vi "SCM1 He level field control.vi"() -> ()   [LabVIEW 2025]
panel:
  out "Waveform Chart":waveform(dbl)(graph)
  in  "level watch dog":bool
  in  "port number":u16=3363
  out "error out":errorcluster
  in  "Data mac ip address":string="146.201.236.102"
  out "low level":bool
  # "Import LHe level from a VI (SCM1 He level.vi) that communicates with the LHe level meter.\nDue to previous issues with communicaiton with the LHe level meter, the SCM1 He level.vi is running in \na separate computer. \nIf the He level is reported to be low, this VI abort some VI's and set the field to zero."
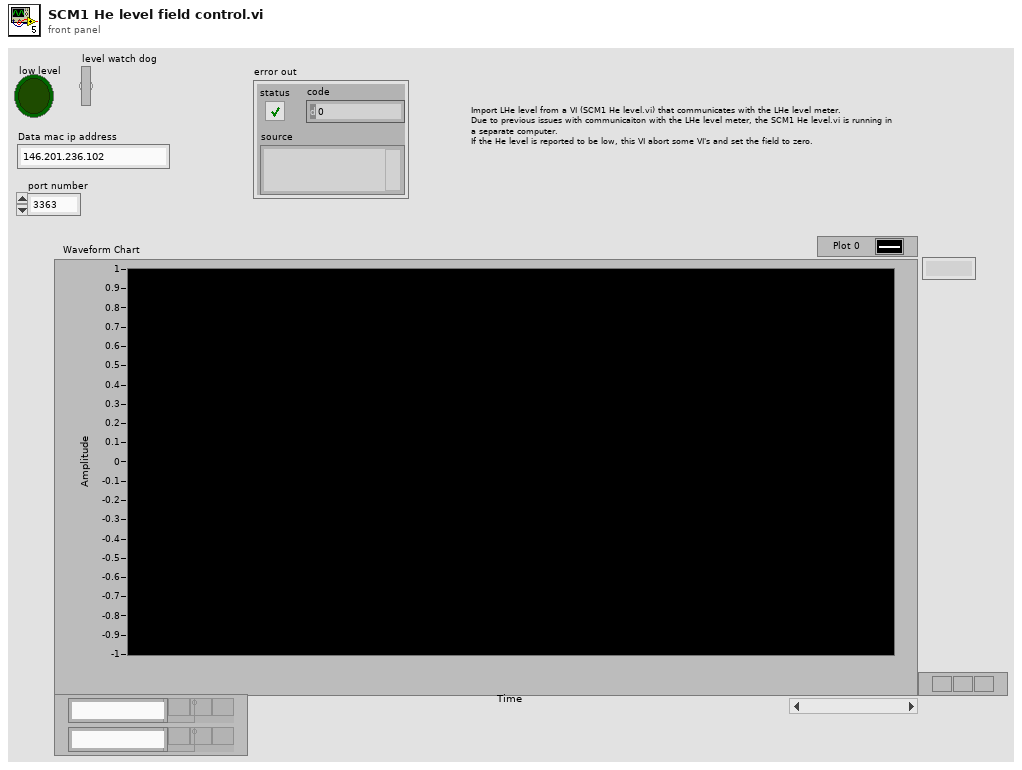
[diagram p1: front panel]
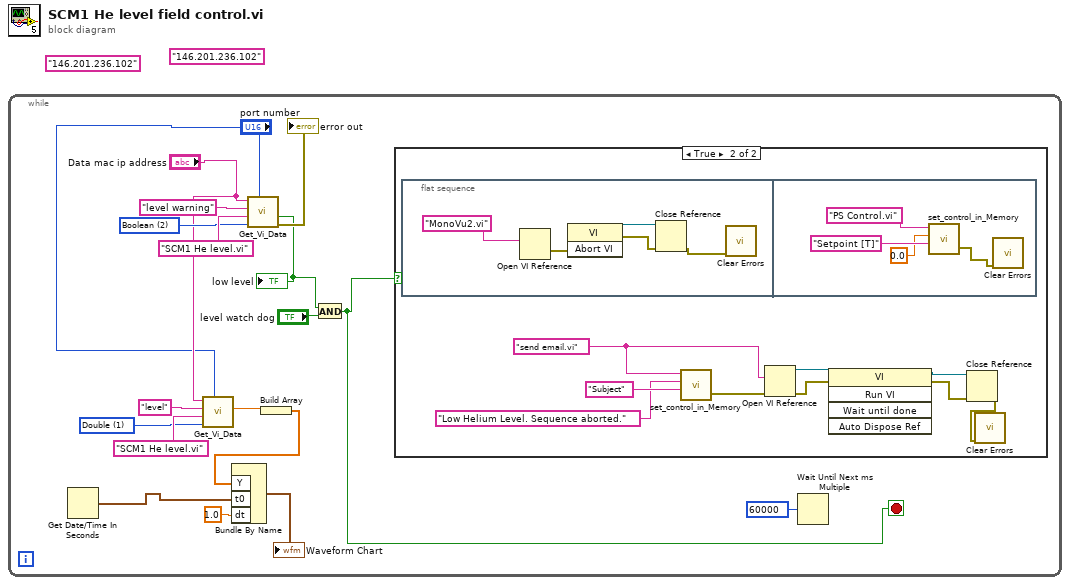
[diagram p0: block diagram]
diagram:
  (unwired) "146.201.236.102" ("Data mac ip address")
  (unwired) "146.201.236.102" ("Data mac ip address")
  n1 = while {
    stop <- w11 stop-if-true
    w8 = u16 1 items=["String", "Double", "Boolean", "Variant"] ("Data Type")
    w15 = u16 2 items=["String", "Double", "Boolean", "Variant"] ("Data Type")
    n2 = Get Date/Time In Seconds() -> (seconds since 1Jan1904=w1:timestamp)
    n3 = call "Get_Vi_Data.vi"("port number"="port number", "Data Type"=w8, "VI name"="SCM1 He level.vi", "Control Name"="level", "Data mac ip address"="Data mac ip address") -> ("Data (Double)"=w4:dbl)  [unwired: 2 in, 4 out]
    n4 = call "Get_Vi_Data.vi"("port number"="port number", "Data Type"=w15, "VI name"="SCM1 He level.vi", "Control Name"="level warning", "Data mac ip address"="Data mac ip address") -> ("error out"=→"error out":errorcluster, "Boolean"=w13:bool)  [unwired: 2 in, 3 out]
    "low level" <- w13
    n5 = Build Array(w4) -> (w3:dbl[])
    n6 = Bundle By Name("Y"=w3, "t0"=w1, "dt"=1.0) -> (→"Waveform Chart":waveform(dbl))  [unwired: 1 in]
    n7 = And(x=w13, y="level watch dog") -> (x .and. y?=w11:bool)
    n8 = case shown="True" w11 {
      frame False {
      }
      frame True {
        w19 = "send email.vi" ("VI Name")
        n9 = flat-sequence {
          frame #0 {
            n10 = Open VI Reference(vi path="MonoVu2.vi" ("VI Name")) -> (error out=w30:errorcluster)  [unwired: 5 in, 1 out]
            n11 = invoke class="VI" method="Abort VI"(error in=w30) -> (reference out=w28:refnum<vi>, error out=w31:errorcluster)  [unwired: 2 in, 1 out]
            n12 = Close Reference(reference=w28, error in (no error)=w31) -> (error out=w32:errorcluster)
            n13 = call <vilib>:"Clear Errors.vi"("error in (no error)"=w32) -> ()  [unwired: 5 in, 2 out]
          }
          frame #1 {
            n14 = call "set_control_in_Memory.vi"("Control Name"="Setpoint [T]", "Value"=0.0 ("y"), "VI Name"="PS Control.vi") -> ("error out 2"=w33:errorcluster)  [unwired: 2 in]
            n15 = call <vilib>:"Clear Errors.vi"("error in (no error)"=w33) -> ()  [unwired: 5 in, 2 out]
          }
        }
        n16 = call "set_control_in_Memory.vi"("Control Name"="Subject", "Value"="Low Helium Level. Sequence aborted." ("Control Name"), "VI Name"=w19) -> ("error out 2"=w20:errorcluster)  [unwired: 2 in]
        n17 = Open VI Reference(vi path=w19, error in (no error)=w20) -> (vi reference=w25:refnum<vi>, error out=w24:errorcluster)  [unwired: 4 in]
        n18 = invoke class="VI" method="Run VI"(reference=w25, error in=w24) -> (reference out=w23:refnum<vi>, error out=w22:errorcluster)  [unwired: 3 in, 3 out]
        n19 = Close Reference(reference=w23, error in (no error)=w22) -> (error out=w21:errorcluster)
        n20 = call <vilib>:"Clear Errors.vi"("error in (no error)"=w21) -> ()  [unwired: 5 in, 2 out]
      }
    }
    n21 = Wait Until Next ms Multiple(millisecond multiple=u32 60000) -> ()  [unwired: 1 out]
  }
